vi "Stop Core.vi"(10 "final error code":i32, 11 "RootModelNotifiesWhenStopped in":refnum<class "ActorNotifiesWhenStopped.lvclass">) -> (3 "RootModelNotifiesWhenStopped out":refnum<class "ActorNotifiesWhenStopped.lvclass">)   [LabVIEW 2017, in "ActorNotifiesWhenStopped.lvclass"]
doc: "(<B>Filename</B>: Actor Framework.lvlib:Actor.lvclass:Stop Core.vi)\n\nDefines what the actor does before it stops. Use the <B>final error code</B> input to determine whether the actor shut down in response to an error.\n\nBy default, this method does nothing. A descendant class may override it to define behavior, such as shutting down any processes the actor initiated in its override of the Actor Core method."
uses:
  ActorNotifiesWhenStopped.lvclass
  ActorNotifiesWhenStopped.lvclass/ActorNotifiesWhenStopped.ctl
  Source/RootModel/RootModel/RootModel.lvclass
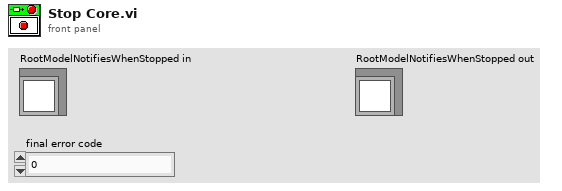
[diagram p1: front panel]
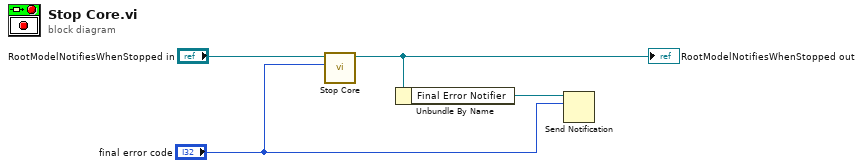
[diagram p0: block diagram]
diagram:
  n1 = call-parent "Stop Core.vi"("final error code"="final error code", "RootModel in"="RootModelNotifiesWhenStopped in") -> ("RootModel out"=w3:refnum<class "ActorNotifiesWhenStopped.lvclass">)  [unwired: 9 in]
  "RootModelNotifiesWhenStopped out" <- w3
  n2 = Unbundle By Name(w3) -> ("Final Error Notifier"=w2:refnum<notifier>)
  n3 = Send Notification(notification="final error code", notifier=w2) -> ()  [unwired: 1 in, 2 out]
